vi "Test3.vi"() -> ()   [LabVIEW 2011]
uses:
  2D_22x22.ctl
panel:
  out "filenames":string[](array[string])
  in  "Boolean 3":T1
  in  "Boolean 2":bool
  in  "Blank Button":bool
  in  "Boolean":bool
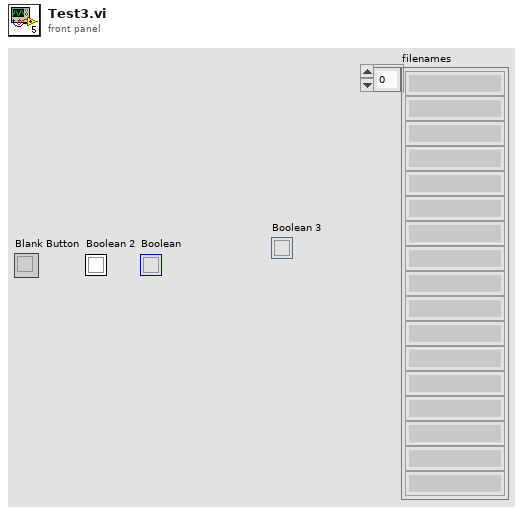
[diagram p1: front panel]
types:
  T1 = typedef "2D_22x22.ctl" = bool
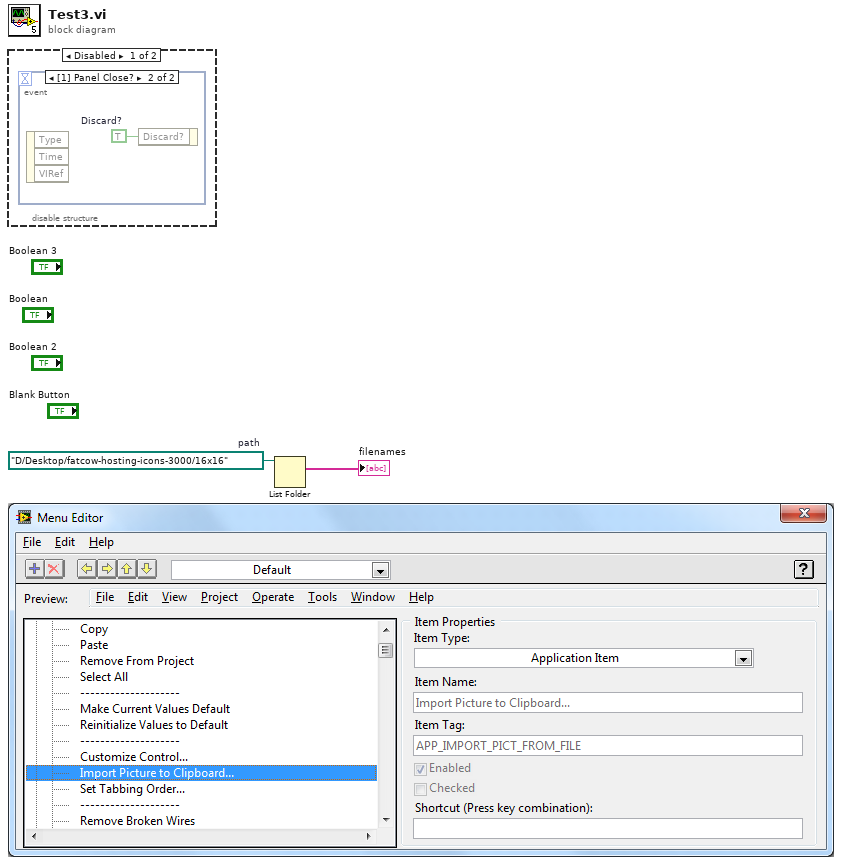
[diagram p0: block diagram]
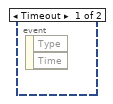
[diagram p2: hidden frame]
diagram:
  w2 = path "D:/Desktop/fatcow-hosting-icons-3000/16x16"  # path
  n1 = disable-structure shown="Disabled" {
    frame Disabled {
      n2 = event shown="[1] Panel Close?" {
        selector: _ -> [_ _]
        dyn-events: _ -> [_ _]
        timeout: _ -> [_ _]
        event Timeout {
          n3 = event-data() -> ()  [unwired: 1 in, 2 out]
        }
        event Panel Close? {
          w3 = TRUE  # Discard?
          n4 = event-data() -> ()  [unwired: 1 in, 3 out]
          n5 = event-data("Discard?"=w3) -> ()  [unwired: 1 in, 1 out]
        }
      }
    }
    frame Enabled {
    }
  }
  n6 = List Folder(path=w2) -> (filenames=→"filenames":string[])  [unwired: 3 in, 3 out]
